vi "Get Library Classes.vi"(8 "error in (no error)":errorcluster, 11 "library ref":refnum<vi>) -> (0 "error out":errorcluster, 2 "class names":string[](array[string]), 3 "class refs":refnum<vi>[](array[refnum]))   [LabVIEW 2020, in "Build Automation.lvlib"]
uses:
  Build Automation.lvlib
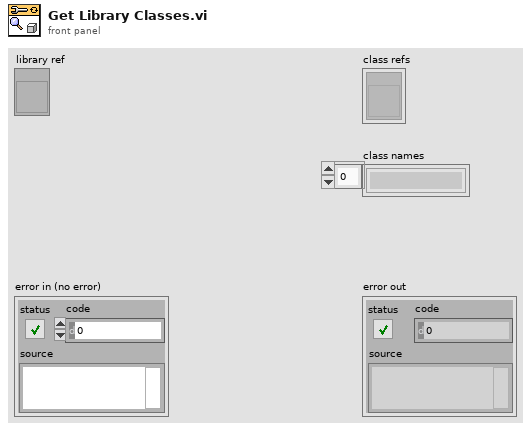
[diagram p1: front panel]
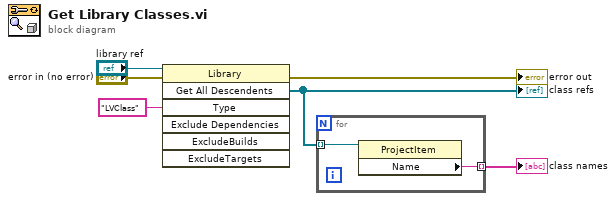
[diagram p0: block diagram]
diagram:
  n1 = invoke class="Library" method="Get All Descendents"(reference="library ref", error in="error in (no error)", "Type"="LVClass" ("y")) -> (error out=→"error out":errorcluster, "All Descendents"=w2:refnum<vi>[])  [unwired: 4 in, 5 out]
  "class refs" <- w2
  n2 = for {
    tunnel: w2 -> [w8] mode=indexing
    tunnel: [w7] -> w1 mode=indexing
    n3 = property class="ProjectItem"(reference=w8) -> ("Name"=w7:string)  [unwired: 1 in, 2 out]
  }
  "class names" <- w1
